vi "GT_SetCrdPrm.vi"(4 "Y":T2=2 items=["Axis Control"=0, "Axis 1"=1, "Axis 2"=2, "Axis 3"=3, "Axis 4"=4, "Axis 5"=5, "Axis 6"=6, "Axis 7"=7, "Axis 8"=8, "Vector Space Control"=16, "Vector Space 1"=17, "Vector Space 2"=18, "Vector Space 3"=19, "Vector Space 4"=20], 6 "X":T2=1 items=["Axis Control"=0, "Axis 1"=1, "Axis 2"=2, "Axis 3"=3, "Axis 4"=4, "Axis 5"=5, "Axis 6"=6, "Axis 7"=7, "Axis 8"=8, "Vector Space Control"=16, "Vector Space 1"=17, "Vector Space 2"=18, "Vector Space 3"=19, "Vector Space 4"=20], 7 "Z":T2 items=["Axis Control"=0, "Axis 1"=1, "Axis 2"=2, "Axis 3"=3, "Axis 4"=4, "Axis 5"=5, "Axis 6"=6, "Axis 7"=7, "Axis 8"=8, "Vector Space Control"=16, "Vector Space 1"=17, "Vector Space 2"=18, "Vector Space 3"=19, "Vector Space 4"=20], 8 "dimension":i16(ring)=2 items=["2 Dimension"=2, "3 Dimension"=3], 9 "pCrdPrm":T3={"synVelMax"=500.0, "synAccMax"=500.0, "evenTime"=50}, 10 "crd":i16=1, 11 "rtn_In":cluster{"rtn":i16, "Func":string}) -> (2 "crd out":i16=1, 3 "rtn_Out":cluster{"rtn":i16, "Func":string})   [LabVIEW 2014]
uses:
  <vilib>/Motion/FlexMotion/CustomControls/CustomControls.llb/AxisOrVectorSpaceControl To Control.flx
  VC6/gts.dll
panel:
  out "输出簇":T1
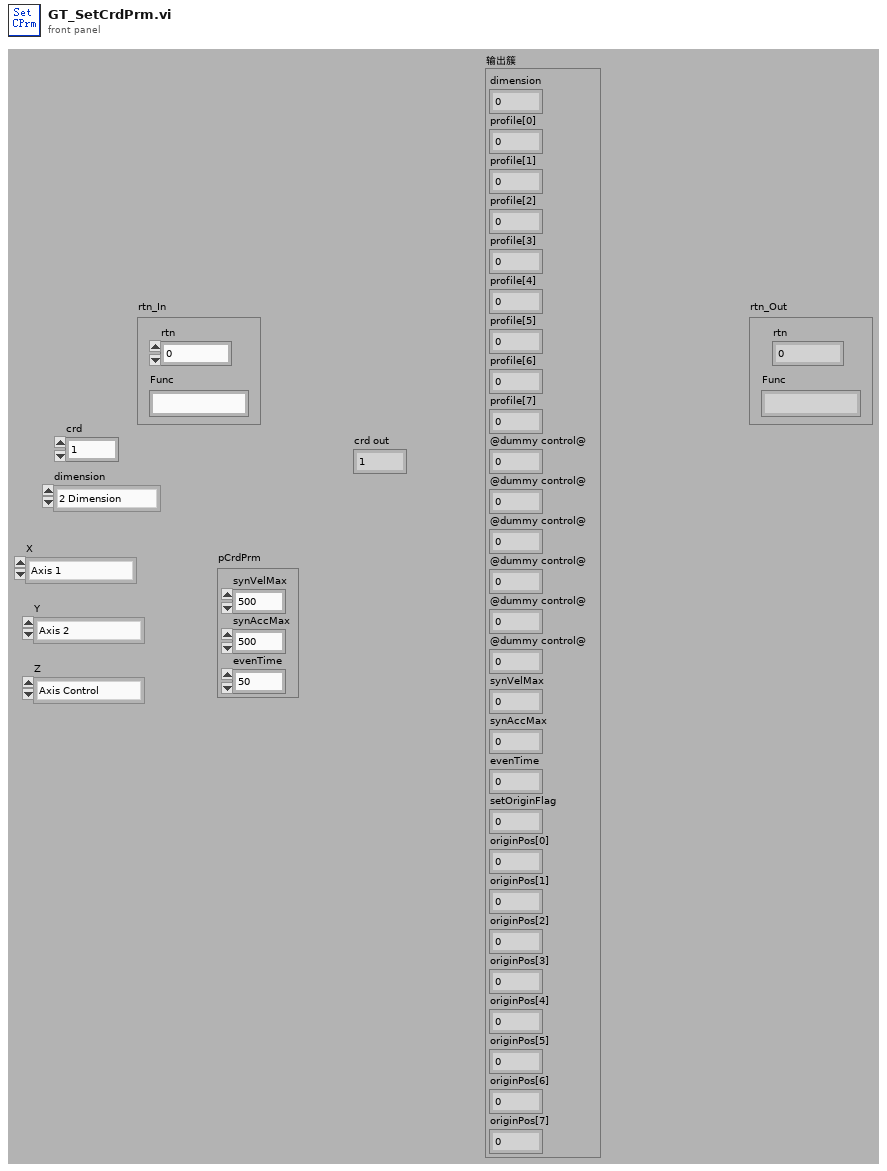
[diagram p1: front panel]
types:
  T1 = cluster{"dimension":i16, "profile[0]":i16, "profile[1]":i16, "profile[2]":i16, "profile[3]":i16, "profile[4]":i16, "profile[5]":i16, "profile[6]":i16, "profile[7]":i16, "@dummy control@":i8, "@dummy control@":i8, "@dummy control@":i8, "@dummy control@":i8, "@dummy control@":i8, "@dummy control@":i8, "synVelMax":dbl, "synAccMax":dbl, "evenTime":i16, "setOriginFlag":i16, "originPos[0]":i32, "originPos[1]":i32, "originPos[2]":i32, "originPos[3]":i32, "originPos[4]":i32, "originPos[5]":i32, "originPos[6]":i32, "originPos[7]":i32}
  T2 = typedef "AxisOrVectorSpaceControl To Control.flx" = u16
  T3 = cluster{"synVelMax":dbl, "synAccMax":dbl, "evenTime":i16}
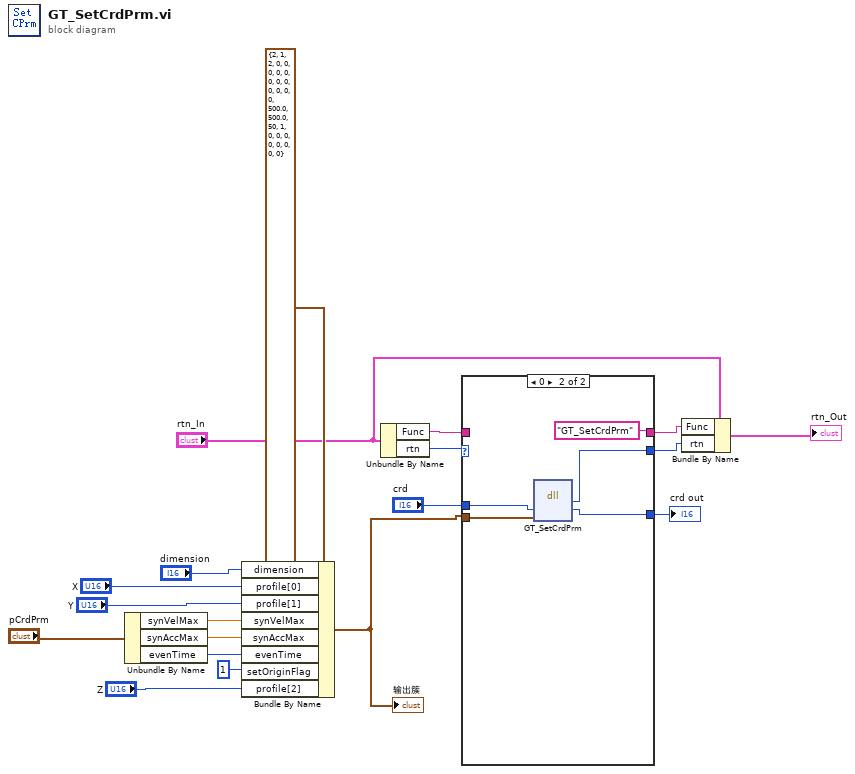
[diagram p0: block diagram]
diagram:
  n1 = Unbundle By Name("pCrdPrm") -> ("synVelMax"=w14:dbl, "synAccMax"=w15:dbl, "evenTime"=w16:i16)
  n2 = Bundle By Name(cluster=T1 {"dimension"=2, "profile[0]"=1, "profile[1]"=2, "profile[2]"=0, "profile[3]"=0, "profile[4]"=0, "profile[5]"=0, "profile[6]"=0, "profile[7]"=0, "@dummy control@"=0, "@dummy control@"=0, "@dummy control@"=0, "@dummy control@"=0, "@dummy control@"=0, "@dummy control@"=0, "synVelMax"=500.0, "synAccMax"=500.0, "evenTime"=50, "setOriginFlag"=1, "originPos[0]"=0, "originPos[1]"=0, "originPos[2]"=0, "originPos[3]"=0, "originPos[4]"=0, "originPos[5]"=0, "originPos[6]"=0, "originPos[7]"=0} ("pCrdPrm 5"), "dimension"="dimension", "profile[0]"="X", "profile[1]"="Y", "synVelMax"=w14, "synAccMax"=w15, "evenTime"=w16, "setOriginFlag"=i16 1, "profile[2]"="Z") -> (w1:T1)
  "输出簇" <- w1
  n3 = Unbundle By Name("rtn_In") -> ("Func"=w9:string, "rtn"=w12:i16)
  n4 = case shown="0" w12 {
    selector: w12 -> [w22 _]
    tunnel: w1 -> [_ w24]
    tunnel: [w22 w27] -> w11
    tunnel: "crd" -> [w21 w26]
    tunnel: [w21 w25] -> w18
    tunnel: [w20 "GT_SetCrdPrm" ("Func")] -> w10
    tunnel: w9 -> [w20 _]
    frame Default {
    }
    frame 0 {
      n5 = dll-call lib="PTH2Fabs DNewGTS AC-800LWin7版源程序-20170926gts85VC6gts.dll" fn="GT_SetCrdPrm"("crd"=w26, "pCrdPrm"=w24) -> ("rtn"=w27:i16, "crd"=w25:i16)  [unwired: 4 in, 2 out]
    }
  }
  "crd out" <- w18
  n6 = Bundle By Name(cluster="rtn_In", "Func"=w10, "rtn"=w11) -> (→"rtn_Out":cluster{"rtn":i16, "Func":string})
